vi "init one data map.vi"(9 "DCAF Type":T2, 10 "Allocations":string[](array[string]), 11 "Data Maps In":T1[](array[typedef])) -> (3 "Data Maps Out":T1[](array[typedef]))   [LabVIEW 2014, in "SQLite runtime.lvclass"]
uses:
  SQLite runtime.lvclass
  <vilib>/NI/Tag Bus/tag/Data Type.ctl
  data map.ctl
  sqlite type.ctl
  <vilib>/NI/Tag Bus/tag/tag descriptor.lvclass
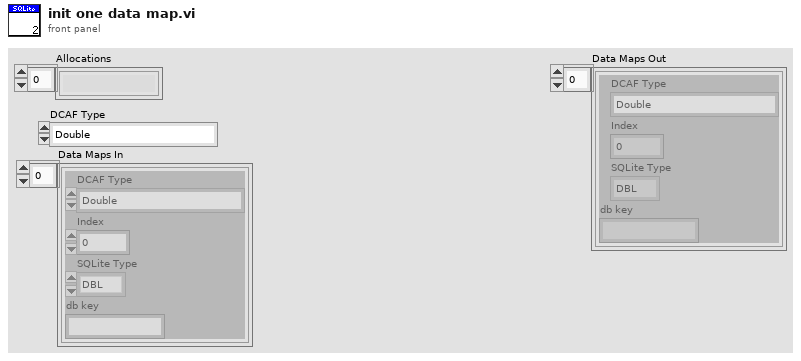
[diagram p1: front panel]
types:
  T1 = typedef "SQLite runtime.lvclass/data map.ctl" = cluster{"DCAF Type":T2, "Index":i32, "SQLite Type":T3, "db key":string}
  T2 = typedef "tag bus.lvlib/tag descriptor.lvclass/Data Type.ctl" = enum16{"Double", "Single", "I64", "I32", "I16", "I8", "U64", "U32", "U16", "U8", "Boolean", "String", "Array of Double", "Array of Single", "Array of I64", "Array of I32", "Array of I16", "Array of I8", "Array of U64", "Array of U32", "Array of U16", "Array of U8", "Array of Boolean", "Array of String"}
  T3 = typedef "SQLite runtime.lvclass/sqlite type.ctl" = enum16{"DBL", "I64", "String"}
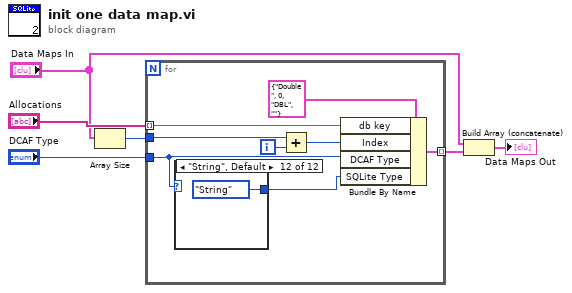
[diagram p0: block diagram]
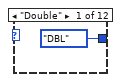
[diagram p2: hidden frame]
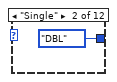
[diagram p3: hidden frame]
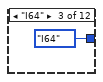
[diagram p4: hidden frame]
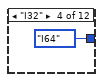
[diagram p5: hidden frame]
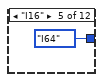
[diagram p6: hidden frame]
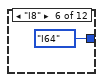
[diagram p7: hidden frame]
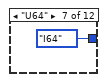
[diagram p8: hidden frame]
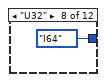
[diagram p9: hidden frame]
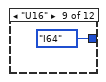
[diagram p10: hidden frame]
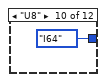
[diagram p11: hidden frame]
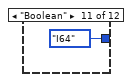
[diagram p12: hidden frame]
diagram:
  n1 = Array Size(array="Data Maps In") -> (size(s)=w4:i32)
  n2 = for {
    tunnel: "Allocations" -> [w10] mode=indexing
    tunnel: "DCAF Type" -> [w8]
    tunnel: [w13] -> w2 mode=indexing
    tunnel: w4 -> [w12]
    i -> [w11]
    n3 = case shown="\"String\", Default" w8 {
      tunnel: [sqlite_type."DBL" ("SQLite Type") sqlite_type."DBL" ("SQLite Type") sqlite_type."I64" ("SQLite Type") sqlite_type."I64" ("SQLite Type") sqlite_type."I64" ("SQLite Type") sqlite_type."I64" ("SQLite Type") sqlite_type."I64" ("SQLite Type") sqlite_type."I64" ("SQLite Type") sqlite_type."I64" ("SQLite Type") sqlite_type."I64" ("SQLite Type") sqlite_type."I64" ("SQLite Type") sqlite_type."String" ("SQLite Type")] -> w7
      frame "Double" {
      }
      frame "Single" {
      }
      frame "I64" {
      }
      frame "I32" {
      }
      frame "I16" {
      }
      frame "I8" {
      }
      frame "U64" {
      }
      frame "U32" {
      }
      frame "U16" {
      }
      frame "U8" {
      }
      frame "Boolean" {
      }
      frame "String", Default {
      }
    }
    n4 = Add(x=w12, y=w11) -> (x+y=w9:i32)
    n5 = Bundle By Name(cluster=T1 {"DCAF Type"=enum."Double", "Index"=0, "SQLite Type"=enum."DBL", "db key"=""} ("Input"), "db key"=w10, "Index"=w9, "DCAF Type"=w8, "SQLite Type"=w7) -> (w13:T1)
  }
  n6 = Build Array (concatenate)("Data Maps In", w2) -> (→"Data Maps Out":T1[])
